vi "Set Check Enabled.vi"(8 "error in (no error)":errorcluster {"code" format="%.0x"}, 9 "ChannelList":string, 10 "Enabled (Off)":bool, 11 "instrument handle":refnum<k15>) -> (0 "error out":errorcluster {"code" format="%.0x"}, 3 "instrument handle out":refnum<k15>)   [LabVIEW 2020, in "Keysight DAQ970.lvlib"]
doc: "Sets the thermocouple check feature state on the specified channelList or current scan list if parameter is empty, to verify the thermocouple is properly connected. If enabled, the instrument measures the channel resistance after each thermocouple measurement to ensure a proper connection. If an open connection is detected (>5 k? on the 10 k? range), the instrument reports an overload condition for that channel's temperature reading."
uses:
  Keysight DAQ970.lvlib
  KtDAQ970.dll
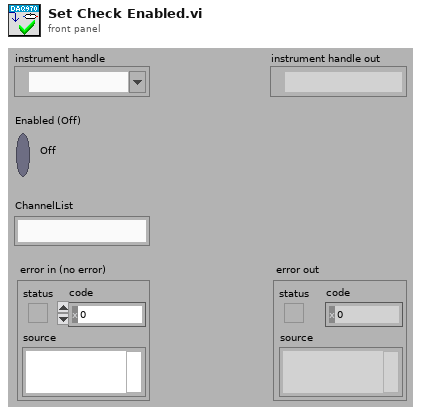
[diagram p1: front panel]
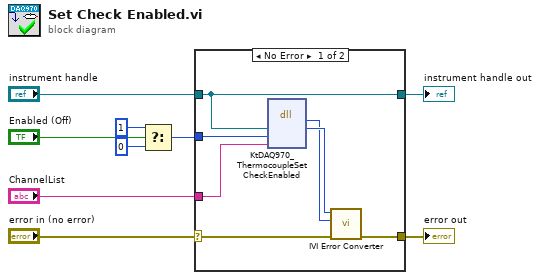
[diagram p0: block diagram]
diagram:
  n1 = Select(t=u16 1, s="Enabled (Off)", f=u16 0) -> (s? t:f=w3:u16)
  n2 = case shown="No Error" "error in (no error)" {
    selector: "error in (no error)" -> [w14 w18]
    tunnel: [w13 w18] -> w9
    tunnel: "instrument handle" -> [w10 w17]
    tunnel: w3 -> [w12 _]
    tunnel: "ChannelList" -> [w11 _]
    tunnel: [w10 w17] -> w1
    frame No Error {
      n3 = dll-call lib="KtDAQ970**.dll" fn="KtDAQ970_ThermocoupleSetCheckEnabled"("Vi"=w10, "Enabled"=w12, "ChannelList"=w11) -> (w15:i32, "Vi"=w16:u32)  [unwired: 5 in, 2 out]
      n4 = call "IVI Error Converter.vi"("error in (no error)"=w14, "IVI error code (0)"=w15, "instrument handle"=w16) -> ("error out"=w13:errorcluster)  [unwired: 7 in, 1 out]
    }
    frame Error {
    }
  }
  "error out" <- w9
  "instrument handle out" <- w1
